vi "Drive Straight Gyro.vi"(8 "PID gains":T1={"proportional gain (Kc)"=0.01, "integral time (Ti, min)"=0.0, "derivative time (Td, min)"=0.0} {"derivative time (Td, min)" format="%.3f"; "integral time (Ti, min)" format="%.3f"; "proportional gain (Kc)" format="%.3f"}, 9 "Process Variable type (Encoders)":enum16{"Encoders", "Vision Distrance"}(ring), 10 "output range":cluster{"output high":dbl, "output low":dbl}={"output high"=0.7, "output low"=-0.7}, 11 "Distance to travel":dbl) -> (3 "In Range?":bool)   [LabVIEW 2015]
uses:
  Robot Values.vi
  <vilib>/addons/control/pid/pid.llb/PID (DBL).vi
  <vilib>/addons/control/pid/NI_PID_pid.lvlib
panel:
  in  "First Call":bool
  in  "Fiirst Call":bool=TRUE
  in  "Gyro PID gains":T1={"proportional gain (Kc)"=0.05, "integral time (Ti, min)"=0.0, "derivative time (Td, min)"=0.0} {"derivative time (Td, min)" format="%.3f"; "integral time (Ti, min)" format="%.3f"; "proportional gain (Kc)" format="%.3f"}
  in  "Tolerance":dbl=20.0
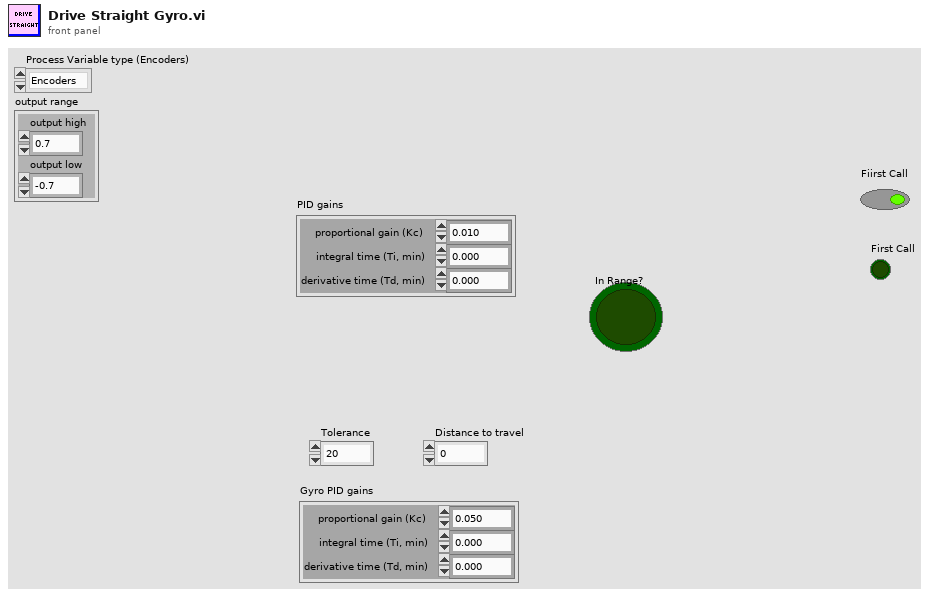
[diagram p1: front panel]
types:
  T1 = cluster{"proportional gain (Kc)":dbl, "integral time (Ti, min)":dbl, "derivative time (Td, min)":dbl}
  T2 = typedef "Robot Values.ctl" = cluster{"Drive Motors":cluster{"Left Motor Value":dbl, "Right Motor Value":dbl, "Left Motor Encoder":dbl, "Right Motor Encoder":dbl, "High/Low Gear":bool}, "Sensors":cluster{"Gyro Angle":dbl, "Photoeye":bool, "Ultrasonic Range":dbl, "Shooter Speed Encoder":dbl, "Accelerometer Value":dbl, "Flashlight":bool, "Target Distance":dbl, "Target X Value":dbl, "Reset Gyro?":bool}, "Arms":cluster{"Desired Arm Position":dbl, "Left Arm Encoder":dbl, "Right Arm Encoder":dbl, "Left Arm Lower Limit":bool, "Right Arm Lower Limit":bool, "Initialize Arm Position?":bool}, "Acquisition and Scoring":cluster{"Acquiring?":bool, "Current Speed":dbl, "Setpoint Speed":dbl, "Prep Wheels":bool, "Shoot":bool, "Low Eject":bool, "Reverse Shooter Wheel":bool}, "Hanging":cluster{"Pivot Arms":dbl, "PTO":bool, "Left Pivot Encoder":dbl, "Right Pivot Encoder":dbl, "Hanging Pin":bool}}
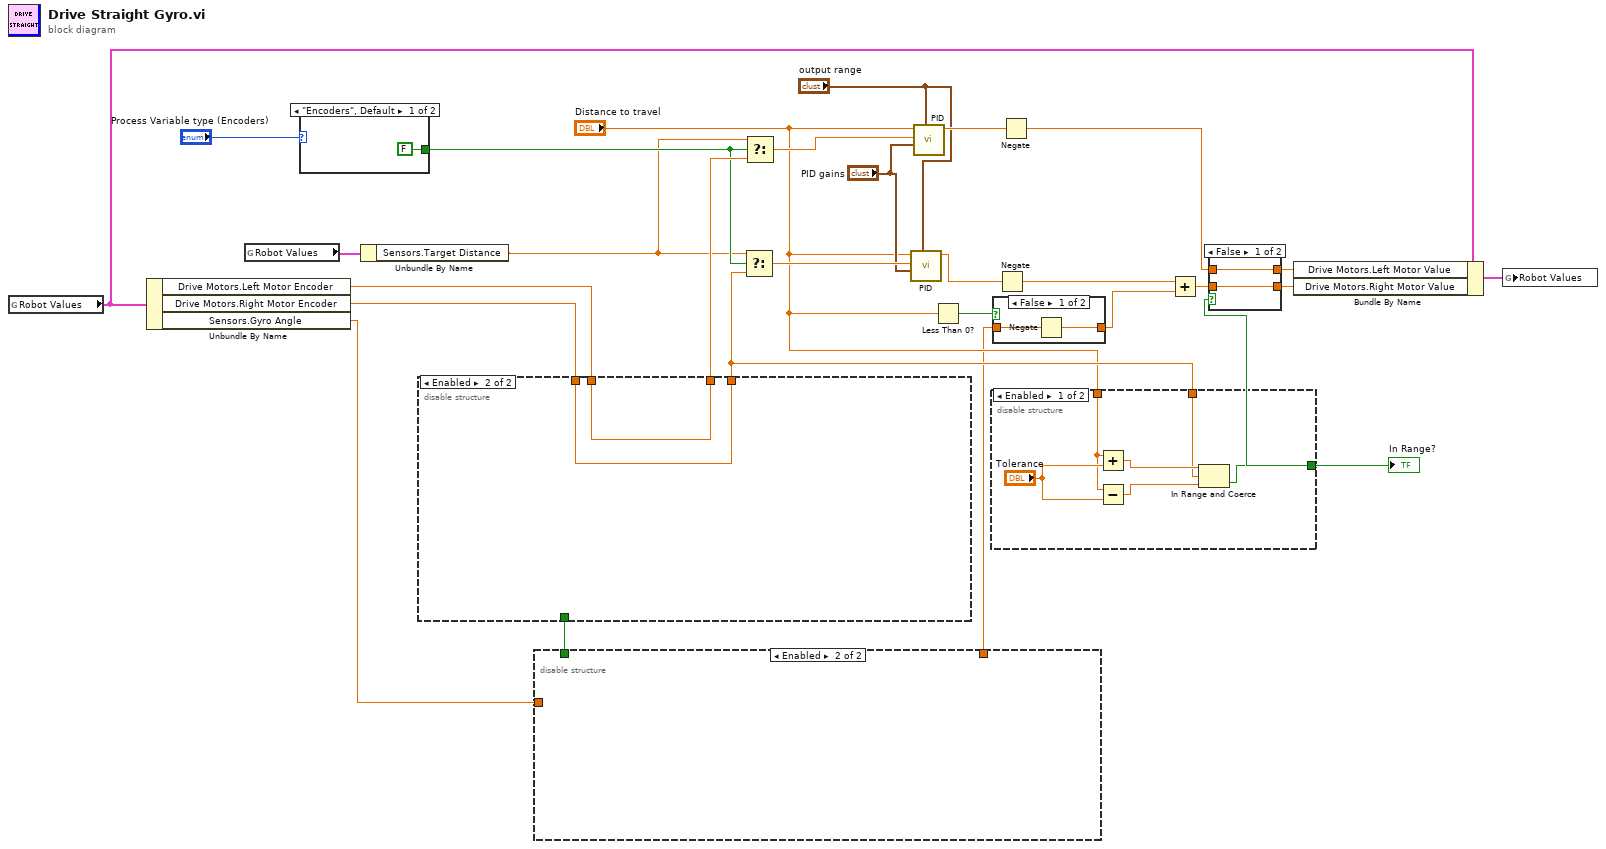
[diagram p0: block diagram]
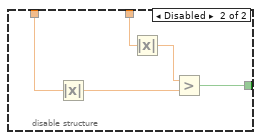
[diagram p3: hidden frame]
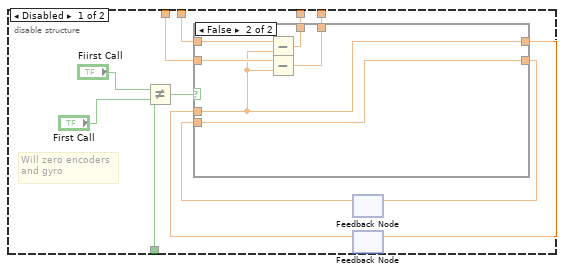
[diagram p4: hidden frame]
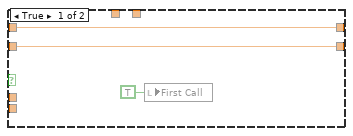
[diagram p5: hidden frame]
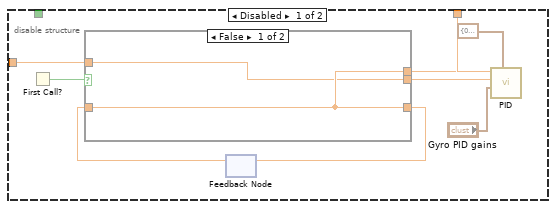
[diagram p6: hidden frame]
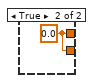
[diagram p8: hidden frame]
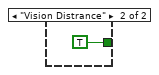
[diagram p9: hidden frame]
diagram:
  n1 = global read "Robot Values.vi" "Robot Values"() -> (w26:T2)
  n2 = Unbundle By Name(w26) -> ("Drive Motors.Left Motor Encoder"=w24:dbl, "Drive Motors.Right Motor Encoder"=w28:dbl, "Sensors.Gyro Angle"=w23:dbl)
  n3 = global read "Robot Values.vi" "Robot Values"() -> (w16:T2)
  n4 = case shown="\"Encoders\", Default" "Process Variable type (Encoders)" {
    tunnel: [FALSE TRUE] -> w18
    frame "Encoders", Default {
    }
    frame "Vision Distrance" {
    }
  }
  n5 = Unbundle By Name(w16) -> ("Sensors.Target Distance"=w15:dbl)
  n6 = disable-structure shown="Enabled" {
    disable-tunnel: w28 -> [w41 w51]
    disable-tunnel: w24 -> [w36 w52]
    disable-tunnel: [w35 w52] -> w21
    disable-tunnel: [w34 w51] -> w14
    disable-tunnel: [w31 _] -> w5
    frame Disabled {
      # "Will zero encoders\nand gyro"
      n7 = Not Equal?(x="Fiirst Call", y="First Call") -> (x != y?=w31:bool)
      n8 = feedback #1() -> (w38:dbl)  [unwired: 1 in]
      n9 = feedback #2() -> (w37:dbl)  [unwired: 1 in]
      n10 = case shown="False" w31 {
        tunnel: w36 -> [w44 w49]
        tunnel: w41 -> [w43 w48]
        tunnel: [w44 w45] -> w39
        tunnel: [w43 w50] -> w40
        tunnel: w38 -> [_ w50]
        tunnel: w37 -> [_ w45]
        tunnel: [_ w47] -> w34
        tunnel: [_ w46] -> w35
        frame True {
          n11 = local write "First Call"(TRUE ("First Call")) -> ()
        }
        frame False {
          n12 = Subtract(x=w49, y=w45) -> (x-y=w46:dbl)
          n13 = Subtract(x=w48, y=w45) -> (x-y=w47:dbl)
        }
      }
      n14 = feedback-in #1(w40) -> ()
      n15 = feedback-in #2(w39) -> ()
    }
    frame Enabled {
    }
  }
  n16 = disable-structure shown="Enabled" {
    disable-tunnel: w5 -> [_ _]
    disable-tunnel: w23 -> [w61 _]
    disable-tunnel: [w56 _] -> w2
    frame Disabled {
      n17 = First Call?() -> (First Call?: T/F=w53:bool)
      n18 = feedback #3() -> (w59:dbl)  [unwired: 1 in]
      n19 = case shown="False" w53 {
        tunnel: w61 -> [w62 w64]
        tunnel: [w63 w64] -> w60
        tunnel: w59 -> [w63 _]
        tunnel: [w63 w64] -> w55
        tunnel: [w62 w64] -> w54
        frame False {
        }
        frame True {
        }
      }
      n20 = feedback-in #3(w60) -> ()
      n21 = call-poly <vilib>:"PID.vi"("output range"=cluster{"output high":dbl, "output low":dbl} {"output high"=0.3, "output low"=-0.3}, "PID gains"="Gyro PID gains", "process variable"=w54, "setpoint"=w55) -> ("output"=w56:dbl)  [unwired: 6 in, 1 out]
    }
    frame Enabled {
    }
  }
  n22 = Select(t=w15, s=w18, f=w14) -> (s? t:f=w22:dbl)
  n23 = Select(t=w15, s=w18, f=w21) -> (s? t:f=w20:dbl)
  n24 = call-poly <vilib>:"PID.vi"("output range"="output range", "PID gains"="PID gains", "process variable"=w22, "setpoint"="Distance to travel") -> ("output"=w17:dbl)  [unwired: 6 in, 1 out]
  n25 = call-poly <vilib>:"PID.vi"("output range"="output range", "PID gains"="PID gains", "process variable"=w20, "setpoint"="Distance to travel") -> ("output"=w25:dbl)  [unwired: 6 in, 1 out]
  n26 = Less Than 0?(x="Distance to travel") -> (x < 0?=w3:bool)
  n27 = disable-structure shown="Enabled" {
    disable-tunnel: "Distance to travel" -> [w69 w74]
    disable-tunnel: w14 -> [w66 w75]
    disable-tunnel: [w65 w73] -> w8
    frame Enabled {
      n28 = Add(x=w69, y="Tolerance") -> (x+y=w68:dbl)
      n29 = Subtract(x=w69, y="Tolerance") -> (x-y=w67:dbl)
      n30 = In Range and Coerce(upper limit=w68, x=w66, lower limit=w67) -> (In Range?=w65:bool)  [unwired: 1 out]
    }
    frame Disabled {
      n31 = Absolute Value(x=w74) -> (abs(x)=w71:dbl)
      n32 = Absolute Value(x=w75) -> (abs(x)=w72:dbl)
      n33 = Greater?(x=w72, y=w71) -> (0:w73:bool)
    }
  }
  "In Range?" <- w8
  n34 = case shown="False" w3 {
    tunnel: w2 -> [w77 w78]
    tunnel: [w76 w78] -> w1
    frame False {
      n35 = Negate(x=w77) -> (-x=w76:dbl)
    }
    frame True {
    }
  }
  n36 = Negate(x=w17) -> (-x=w13:dbl)
  n37 = Negate(x=w25) -> (-x=w12:dbl)
  n38 = Add(x=w13, y=w1) -> (x+y=w11:dbl)
  n39 = case shown="False" w8 {
    tunnel: w12 -> [w79 _]
    tunnel: w11 -> [w80 _]
    tunnel: [w80 w81] -> w10
    tunnel: [w79 w81] -> w9
    frame False {
    }
    frame True {
      w81 = 0.0
    }
  }
  n40 = Bundle By Name(cluster=w26, "Drive Motors.Left Motor Value"=w9, "Drive Motors.Right Motor Value"=w10) -> (w27:T2)
  n41 = global write "Robot Values.vi" "Robot Values"(w27) -> ()
